vi "Bands_Main.vi"() -> ()   [LabVIEW 2024]
panel:
  out "Band sdev":dbl[][](graph)=[[0.3353772546826648, 0.4084966641388683, 0.5003856797342301, 0.6478785546391153], [0.24171080418296995, 0.35230228586245604, 0.3759732028560709, 0.5033028137104077], [0.22150470046762238, 0.3310214612014374, 0.36292977087510636, 0.4846104192263559], [0.19277937218238525, 0.3163483721041411, 0.36220368337093534, 0.46553114605932655], [0.19710471438384322, 0.32700679595860704, 0.3029446613190426, 0.4492463332131647], [0.16819270542381565, 0.31656348385339184, 0.35242193549705353, 0.427055332660449], [0.1730511001135913, 0.3123187705631996, 0.28252942293417965, 0.4121174290079004], [0.18605777226992246, 0.3065454715716774, 0.30903285463424796, 0.4641767502949591], [0.16818659712668763, 0.2724970239281444, 0.3555985592674683, 0.44590883736070325], [0.16166367655910485, 0.3076354897837717, 0.1949896816550948, 0.425321351327427], [0.14596500451769295, 0.2564716293467485, 0.3273362893696218, 0.44524121627082514], [0.1522592511319178, 0.29229701933526936, 0.22508584133149354, 0.44741414361442283], [0.14416764010644756, 0.28551749160160084, 0.27379096985814816, 0.4513185261438864], [0.17394046024499085, 0.27596830396614264, 0.3207441771446193, 0.451484391576808], [0.18167741119745937, 0.3045239509747764, 0.3000903307112586, 0.4481452184981623]]
  out "Band averages":dbl[][](graph)=[[8.680626893486426, 8.606188361284897, 12.33777384261614, 8.164276802226652], [8.632200271675586, 8.585758096325415, 12.307413887785566, 8.160446575120634], [8.624357532912756, 8.586135493161098, 12.319276005863179, 8.180110072455836], [8.616888139440022, 8.595026675175392, 12.33629120572369, 8.226922143493606], [8.616565415492165, 8.584035276166606, 12.32246082387115, 8.229027322702942], [8.62061301332379, 8.596221440305454, 12.351044023184894, 8.232899394943033], [8.617026039579283, 8.600839570954378, 12.356456884526148, 8.263498869003483], [8.624746125158572, 8.602677323174724, 12.37154176572413, 8.278567915663922], [8.612707346903331, 8.608183345601441, 12.400573947592072, 8.284231055046059], [8.610867167958734, 8.600263543620425, 12.357185805915336, 8.27523640312406], [8.60675426215495, 8.601551581496466, 12.40037793823958, 8.277235304213152], [8.613147504083752, 8.59805082398266, 12.383603489290671, 8.29105542356648], [8.621277473998088, 8.594195350754449, 12.433606127342339, 8.341301392017439], [8.617604109548608, 8.618650848461376, 12.428611676476121, 8.316097099348083], [8.635651626479794, 8.611122304003379, 12.453260394927339, 8.37908607476574]]
  in  "Bands 2":u16(ring)=2 items=["No Bands", "JC violin 200-7000 Flat (200-7000)", "JC violin (200-780-1740-2930-7000)", "JC violin (200-780-7000)", "MJ_Test (200-428-453-780-1740-2930-7000)"]
  in  "Files":path[](array[path])=[path "/Users/crogers/Dropbox (Rogers)/Violin Stuff/PC ViolnData/SoundCard2/SoundCard2 ModalShop7/Raw/SoundCard2 ModalShop7 H_001_001.wfm", path "/Users/crogers/Dropbox (Rogers)/Violin Stuff/PC ViolnData/SoundCard2/SoundCard2 ModalShop7/Raw/SoundCard2 ModalShop7 H_001_002.wfm", path "/Users/crogers/Dropbox (Rogers)/Violin Stuff/PC ViolnData/SoundCard2/SoundCard2 ModalShop7/Raw/SoundCard2 ModalShop7 H_001_003.wfm", path "/Users/crogers/Dropbox (Rogers)/Violin Stuff/PC ViolnData/SoundCard2/SoundCard2 ModalShop7/Raw/SoundCard2 ModalShop7 H_001_004.wfm", path "/Users/crogers/Dropbox (Rogers)/Violin Stuff/PC ViolnData/SoundCard2/SoundCard2 ModalShop7/Raw/SoundCard2 ModalShop7 H_001_005.wfm", path "/Users/crogers/Dropbox (Rogers)/Violin Stuff/PC ViolnData/SoundCard2/SoundCard2 ModalShop7/Raw/SoundCard2 ModalShop7 H_001_006.wfm", path "/Users/crogers/Dropbox (Rogers)/Violin Stuff/PC ViolnData/SoundCard2/SoundCard2 ModalShop7/Raw/SoundCard2 ModalShop7 H_001_007.wfm", path "/Users/crogers/Dropbox (Rogers)/Violin Stuff/PC ViolnData/SoundCard2/SoundCard2 ModalShop7/Raw/SoundCard2 ModalShop7 H_001_008.wfm", path "/Users/crogers/Dropbox (Rogers)/Violin Stuff/PC ViolnData/SoundCard2/SoundCard2 ModalShop7/Raw/SoundCard2 ModalShop7 H_001_009.wfm", path "/Users/crogers/Dropbox (Rogers)/Violin Stuff/PC ViolnData/SoundCard2/SoundCard2 ModalShop7/Raw/SoundCard2 ModalShop7 H_001_010.wfm", path "/Users/crogers/Dropbox (Rogers)/Violin Stuff/PC ViolnData/SoundCard2/SoundCard2 ModalShop7/Raw/SoundCard2 ModalShop7 H_002_001.wfm", path "/Users/crogers/Dropbox (Rogers)/Violin Stuff/PC ViolnData/SoundCard2/SoundCard2 ModalShop7/Raw/SoundCard2 ModalShop7 H_002_002.wfm", path "/Users/crogers/Dropbox (Rogers)/Violin Stuff/PC ViolnData/SoundCard2/SoundCard2 ModalShop7/Raw/SoundCard2 ModalShop7 H_002_003.wfm", path "/Users/crogers/Dropbox (Rogers)/Violin Stuff/PC ViolnData/SoundCard2/SoundCard2 ModalShop7/Raw/SoundCard2 ModalShop7 H_002_004.wfm", path "/Users/crogers/Dropbox (Rogers)/Violin Stuff/PC ViolnData/SoundCard2/SoundCard2 ModalShop7/Raw/SoundCard2 ModalShop7 H_002_005.wfm", path "/Users/crogers/Dropbox (Rogers)/Violin Stuff/PC ViolnData/SoundCard2/SoundCard2 ModalShop7/Raw/SoundCard2 ModalShop7 H_002_006.wfm", path "/Users/crogers/Dropbox (Rogers)/Violin Stuff/PC ViolnData/SoundCard2/SoundCard2 ModalShop7/Raw/SoundCard2 ModalShop7 H_002_007.wfm", path "/Users/crogers/Dropbox (Rogers)/Violin Stuff/PC ViolnData/SoundCard2/SoundCard2 ModalShop7/Raw/SoundCard2 ModalShop7 H_002_008.wfm", path "/Users/crogers/Dropbox (Rogers)/Violin Stuff/PC ViolnData/SoundCard2/SoundCard2 ModalShop7/Raw/SoundCard2 ModalShop7 H_002_009.wfm", path "/Users/crogers/Dropbox (Rogers)/Violin Stuff/PC ViolnData/SoundCard2/SoundCard2 ModalShop7/Raw/SoundCard2 ModalShop7 H_002_010.wfm", path "/Users/crogers/Dropbox (Rogers)/Violin Stuff/PC ViolnData/SoundCard2/SoundCard2 ModalShop7/Raw/SoundCard2 ModalShop7 H_003_001.wfm", path "/Users/crogers/Dropbox (Rogers)/Violin Stuff/PC ViolnData/SoundCard2/SoundCard2 ModalShop7/Raw/SoundCard2 ModalShop7 H_003_002.wfm", path "/Users/crogers/Dropbox (Rogers)/Violin Stuff/PC ViolnData/SoundCard2/SoundCard2 ModalShop7/Raw/SoundCard2 ModalShop7 H_003_003.wfm", path "/Users/crogers/Dropbox (Rogers)/Violin Stuff/PC ViolnData/SoundCard2/SoundCard2 ModalShop7/Raw/SoundCard2 ModalShop7 H_003_004.wfm", path "/Users/crogers/Dropbox (Rogers)/Violin Stuff/PC ViolnData/SoundCard2/SoundCard2 ModalShop7/Raw/SoundCard2 ModalShop7 H_003_005.wfm", path "/Users/crogers/Dropbox (Rogers)/Violin Stuff/PC ViolnData/SoundCard2/SoundCard2 ModalShop7/Raw/SoundCard2 ModalShop7 H_003_006.wfm", path "/Users/crogers/Dropbox (Rogers)/Violin Stuff/PC ViolnData/SoundCard2/SoundCard2 ModalShop7/Raw/SoundCard2 ModalShop7 H_003_007.wfm", path "/Users/crogers/Dropbox (Rogers)/Violin Stuff/PC ViolnData/SoundCard2/SoundCard2 ModalShop7/Raw/SoundCard2 ModalShop7 H_003_008.wfm", path "/Users/crogers/Dropbox (Rogers)/Violin Stuff/PC ViolnData/SoundCard2/SoundCard2 ModalShop7/Raw/SoundCard2 ModalShop7 H_003_009.wfm", path "/Users/crogers/Dropbox (Rogers)/Violin Stuff/PC ViolnData/SoundCard2/SoundCard2 ModalShop7/Raw/SoundCard2 ModalShop7 H_003_010.wfm", path "/Users/crogers/Dropbox (Rogers)/Violin Stuff/PC ViolnData/SoundCard2/SoundCard2 ModalShop7/Raw/SoundCard2 ModalShop7 H_004_001.wfm", path "/Users/crogers/Dropbox (Rogers)/Violin Stuff/PC ViolnData/SoundCard2/SoundCard2 ModalShop7/Raw/SoundCard2 ModalShop7 H_004_002.wfm", path "/Users/crogers/Dropbox (Rogers)/Violin Stuff/PC ViolnData/SoundCard2/SoundCard2 ModalShop7/Raw/SoundCard2 ModalShop7 H_004_003.wfm", path "/Users/crogers/Dropbox (Rogers)/Violin Stuff/PC ViolnData/SoundCard2/SoundCard2 ModalShop7/Raw/SoundCard2 ModalShop7 H_004_004.wfm", path "/Users/crogers/Dropbox (Rogers)/Violin Stuff/PC ViolnData/SoundCard2/SoundCard2 ModalShop7/Raw/SoundCard2 ModalShop7 H_004_005.wfm", path "/Users/crogers/Dropbox (Rogers)/Violin Stuff/PC ViolnData/SoundCard2/SoundCard2 ModalShop7/Raw/SoundCard2 ModalShop7 H_004_006.wfm", path "/Users/crogers/Dropbox (Rogers)/Violin Stuff/PC ViolnData/SoundCard2/SoundCard2 ModalShop7/Raw/SoundCard2 ModalShop7 H_004_007.wfm", path "/Users/crogers/Dropbox (Rogers)/Violin Stuff/PC ViolnData/SoundCard2/SoundCard2 ModalShop7/Raw/SoundCard2 ModalShop7 H_004_008.wfm", path "/Users/crogers/Dropbox (Rogers)/Violin Stuff/PC ViolnData/SoundCard2/SoundCard2 ModalShop7/Raw/SoundCard2 ModalShop7 H_004_009.wfm", path "/Users/crogers/Dropbox (Rogers)/Violin Stuff/PC ViolnData/SoundCard2/SoundCard2 ModalShop7/Raw/SoundCard2 ModalShop7 H_004_010.wfm", path "/Users/crogers/Dropbox (Rogers)/Violin Stuff/PC ViolnData/SoundCard2/SoundCard2 ModalShop7/Raw/SoundCard2 ModalShop7 H_005_001.wfm", path "/Users/crogers/Dropbox (Rogers)/Violin Stuff/PC ViolnData/SoundCard2/SoundCard2 ModalShop7/Raw/SoundCard2 ModalShop7 H_005_002.wfm", path "/Users/crogers/Dropbox (Rogers)/Violin Stuff/PC ViolnData/SoundCard2/SoundCard2 ModalShop7/Raw/SoundCard2 ModalShop7 H_005_003.wfm", path "/Users/crogers/Dropbox (Rogers)/Violin Stuff/PC ViolnData/SoundCard2/SoundCard2 ModalShop7/Raw/SoundCard2 ModalShop7 H_005_004.wfm", path "/Users/crogers/Dropbox (Rogers)/Violin Stuff/PC ViolnData/SoundCard2/SoundCard2 ModalShop7/Raw/SoundCard2 ModalShop7 H_005_005.wfm", path "/Users/crogers/Dropbox (Rogers)/Violin Stuff/PC ViolnData/SoundCard2/SoundCard2 ModalShop7/Raw/SoundCard2 ModalShop7 H_005_006.wfm", path "/Users/crogers/Dropbox (Rogers)/Violin Stuff/PC ViolnData/SoundCard2/SoundCard2 ModalShop7/Raw/SoundCard2 ModalShop7 H_005_007.wfm", path "/Users/crogers/Dropbox (Rogers)/Violin Stuff/PC ViolnData/SoundCard2/SoundCard2 ModalShop7/Raw/SoundCard2 ModalShop7 H_005_008.wfm", path "/Users/crogers/Dropbox (Rogers)/Violin Stuff/PC ViolnData/SoundCard2/SoundCard2 ModalShop7/Raw/SoundCard2 ModalShop7 H_005_009.wfm", path "/Users/crogers/Dropbox (Rogers)/Violin Stuff/PC ViolnData/SoundCard2/SoundCard2 ModalShop7/Raw/SoundCard2 ModalShop7 H_005_010.wfm", path "/Users/crogers/Dropbox (Rogers)/Violin Stuff/PC ViolnData/SoundCard2/SoundCard2 ModalShop8/Raw/SoundCard2 ModalShop8 H_001_001.wfm", path "/Users/crogers/Dropbox (Rogers)/Violin Stuff/PC ViolnData/SoundCard2/SoundCard2 ModalShop8/Raw/SoundCard2 ModalShop8 H_001_002.wfm", path "/Users/crogers/Dropbox (Rogers)/Violin Stuff/PC ViolnData/SoundCard2/SoundCard2 ModalShop8/Raw/SoundCard2 ModalShop8 H_001_003.wfm", path "/Users/crogers/Dropbox (Rogers)/Violin Stuff/PC ViolnData/SoundCard2/SoundCard2 ModalShop8/Raw/SoundCard2 ModalShop8 H_001_004.wfm", path "/Users/crogers/Dropbox (Rogers)/Violin Stuff/PC ViolnData/SoundCard2/SoundCard2 ModalShop8/Raw/SoundCard2 ModalShop8 H_001_005.wfm", path "/Users/crogers/Dropbox (Rogers)/Violin Stuff/PC ViolnData/SoundCard2/SoundCard2 ModalShop8/Raw/SoundCard2 ModalShop8 H_001_006.wfm", path "/Users/crogers/Dropbox (Rogers)/Violin Stuff/PC ViolnData/SoundCard2/SoundCard2 ModalShop8/Raw/SoundCard2 ModalShop8 H_001_007.wfm", path "/Users/crogers/Dropbox (Rogers)/Violin Stuff/PC ViolnData/SoundCard2/SoundCard2 ModalShop8/Raw/SoundCard2 ModalShop8 H_001_008.wfm", path "/Users/crogers/Dropbox (Rogers)/Violin Stuff/PC ViolnData/SoundCard2/SoundCard2 ModalShop8/Raw/SoundCard2 ModalShop8 H_001_009.wfm", path "/Users/crogers/Dropbox (Rogers)/Violin Stuff/PC ViolnData/SoundCard2/SoundCard2 ModalShop8/Raw/SoundCard2 ModalShop8 H_001_010.wfm", path "/Users/crogers/Dropbox (Rogers)/Violin Stuff/PC ViolnData/SoundCard2/SoundCard2 ModalShop8/Raw/SoundCard2 ModalShop8 H_002_001.wfm", path "/Users/crogers/Dropbox (Rogers)/Violin Stuff/PC ViolnData/SoundCard2/SoundCard2 ModalShop8/Raw/SoundCard2 ModalShop8 H_002_002.wfm", path "/Users/crogers/Dropbox (Rogers)/Violin Stuff/PC ViolnData/SoundCard2/SoundCard2 ModalShop8/Raw/SoundCard2 ModalShop8 H_002_003.wfm", path "/Users/crogers/Dropbox (Rogers)/Violin Stuff/PC ViolnData/SoundCard2/SoundCard2 ModalShop8/Raw/SoundCard2 ModalShop8 H_002_004.wfm", path "/Users/crogers/Dropbox (Rogers)/Violin Stuff/PC ViolnData/SoundCard2/SoundCard2 ModalShop8/Raw/SoundCard2 ModalShop8 H_002_005.wfm", path "/Users/crogers/Dropbox (Rogers)/Violin Stuff/PC ViolnData/SoundCard2/SoundCard2 ModalShop8/Raw/SoundCard2 ModalShop8 H_002_006.wfm", path "/Users/crogers/Dropbox (Rogers)/Violin Stuff/PC ViolnData/SoundCard2/SoundCard2 ModalShop8/Raw/SoundCard2 ModalShop8 H_002_007.wfm", path "/Users/crogers/Dropbox (Rogers)/Violin Stuff/PC ViolnData/SoundCard2/SoundCard2 ModalShop8/Raw/SoundCard2 ModalShop8 H_002_008.wfm", path "/Users/crogers/Dropbox (Rogers)/Violin Stuff/PC ViolnData/SoundCard2/SoundCard2 ModalShop8/Raw/SoundCard2 ModalShop8 H_002_009.wfm", path "/Users/crogers/Dropbox (Rogers)/Violin Stuff/PC ViolnData/SoundCard2/SoundCard2 ModalShop8/Raw/SoundCard2 ModalShop8 H_002_010.wfm", path "/Users/crogers/Dropbox (Rogers)/Violin Stuff/PC ViolnData/SoundCard2/SoundCard2 ModalShop8/Raw/SoundCard2 ModalShop8 H_003_001.wfm", path "/Users/crogers/Dropbox (Rogers)/Violin Stuff/PC ViolnData/SoundCard2/SoundCard2 ModalShop8/Raw/SoundCard2 ModalShop8 H_003_002.wfm", path "/Users/crogers/Dropbox (Rogers)/Violin Stuff/PC ViolnData/SoundCard2/SoundCard2 ModalShop8/Raw/SoundCard2 ModalShop8 H_003_003.wfm", path "/Users/crogers/Dropbox (Rogers)/Violin Stuff/PC ViolnData/SoundCard2/SoundCard2 ModalShop8/Raw/SoundCard2 ModalShop8 H_003_004.wfm", path "/Users/crogers/Dropbox (Rogers)/Violin Stuff/PC ViolnData/SoundCard2/SoundCard2 ModalShop8/Raw/SoundCard2 ModalShop8 H_003_005.wfm", path "/Users/crogers/Dropbox (Rogers)/Violin Stuff/PC ViolnData/SoundCard2/SoundCard2 ModalShop8/Raw/SoundCard2 ModalShop8 H_003_006.wfm", path "/Users/crogers/Dropbox (Rogers)/Violin Stuff/PC ViolnData/SoundCard2/SoundCard2 ModalShop8/Raw/SoundCard2 ModalShop8 H_003_007.wfm", path "/Users/crogers/Dropbox (Rogers)/Violin Stuff/PC ViolnData/SoundCard2/SoundCard2 ModalShop8/Raw/SoundCard2 ModalShop8 H_003_008.wfm", path "/Users/crogers/Dropbox (Rogers)/Violin Stuff/PC ViolnData/SoundCard2/SoundCard2 ModalShop8/Raw/SoundCard2 ModalShop8 H_003_009.wfm", path "/Users/crogers/Dropbox (Rogers)/Violin Stuff/PC ViolnData/SoundCard2/SoundCard2 ModalShop8/Raw/SoundCard2 ModalShop8 H_003_010.wfm", path "/Users/crogers/Dropbox (Rogers)/Violin Stuff/PC ViolnData/SoundCard2/SoundCard2 ModalShop8/Raw/SoundCard2 ModalShop8 H_004_001.wfm", path "/Users/crogers/Dropbox (Rogers)/Violin Stuff/PC ViolnData/SoundCard2/SoundCard2 ModalShop8/Raw/SoundCard2 ModalShop8 H_004_002.wfm", path "/Users/crogers/Dropbox (Rogers)/Violin Stuff/PC ViolnData/SoundCard2/SoundCard2 ModalShop8/Raw/SoundCard2 ModalShop8 H_004_003.wfm", path "/Users/crogers/Dropbox (Rogers)/Violin Stuff/PC ViolnData/SoundCard2/SoundCard2 ModalShop8/Raw/SoundCard2 ModalShop8 H_004_004.wfm", path "/Users/crogers/Dropbox (Rogers)/Violin Stuff/PC ViolnData/SoundCard2/SoundCard2 ModalShop8/Raw/SoundCard2 ModalShop8 H_004_005.wfm", path "/Users/crogers/Dropbox (Rogers)/Violin Stuff/PC ViolnData/SoundCard2/SoundCard2 ModalShop8/Raw/SoundCard2 ModalShop8 H_004_006.wfm", path "/Users/crogers/Dropbox (Rogers)/Violin Stuff/PC ViolnData/SoundCard2/SoundCard2 ModalShop8/Raw/SoundCard2 ModalShop8 H_004_007.wfm", path "/Users/crogers/Dropbox (Rogers)/Violin Stuff/PC ViolnData/SoundCard2/SoundCard2 ModalShop8/Raw/SoundCard2 ModalShop8 H_004_008.wfm", path "/Users/crogers/Dropbox (Rogers)/Violin Stuff/PC ViolnData/SoundCard2/SoundCard2 ModalShop8/Raw/SoundCard2 ModalShop8 H_004_009.wfm", path "/Users/crogers/Dropbox (Rogers)/Violin Stuff/PC ViolnData/SoundCard2/SoundCard2 ModalShop8/Raw/SoundCard2 ModalShop8 H_004_010.wfm", path "/Users/crogers/Dropbox (Rogers)/Violin Stuff/PC ViolnData/SoundCard2/SoundCard2 ModalShop8/Raw/SoundCard2 ModalShop8 H_005_001.wfm", path "/Users/crogers/Dropbox (Rogers)/Violin Stuff/PC ViolnData/SoundCard2/SoundCard2 ModalShop8/Raw/SoundCard2 ModalShop8 H_005_002.wfm", path "/Users/crogers/Dropbox (Rogers)/Violin Stuff/PC ViolnData/SoundCard2/SoundCard2 ModalShop8/Raw/SoundCard2 ModalShop8 H_005_003.wfm", path "/Users/crogers/Dropbox (Rogers)/Violin Stuff/PC ViolnData/SoundCard2/SoundCard2 ModalShop8/Raw/SoundCard2 ModalShop8 H_005_004.wfm", path "/Users/crogers/Dropbox (Rogers)/Violin Stuff/PC ViolnData/SoundCard2/SoundCard2 ModalShop8/Raw/SoundCard2 ModalShop8 H_005_005.wfm", path "/Users/crogers/Dropbox (Rogers)/Violin Stuff/PC ViolnData/SoundCard2/SoundCard2 ModalShop8/Raw/SoundCard2 ModalShop8 H_005_006.wfm", path "/Users/crogers/Dropbox (Rogers)/Violin Stuff/PC ViolnData/SoundCard2/SoundCard2 ModalShop8/Raw/SoundCard2 ModalShop8 H_005_007.wfm", path "/Users/crogers/Dropbox (Rogers)/Violin Stuff/PC ViolnData/SoundCard2/SoundCard2 ModalShop8/Raw/SoundCard2 ModalShop8 H_005_008.wfm", path "/Users/crogers/Dropbox (Rogers)/Violin Stuff/PC ViolnData/SoundCard2/SoundCard2 ModalShop8/Raw/SoundCard2 ModalShop8 H_005_009.wfm", path "/Users/crogers/Dropbox (Rogers)/Violin Stuff/PC ViolnData/SoundCard2/SoundCard2 ModalShop8/Raw/SoundCard2 ModalShop8 H_005_010.wfm"]
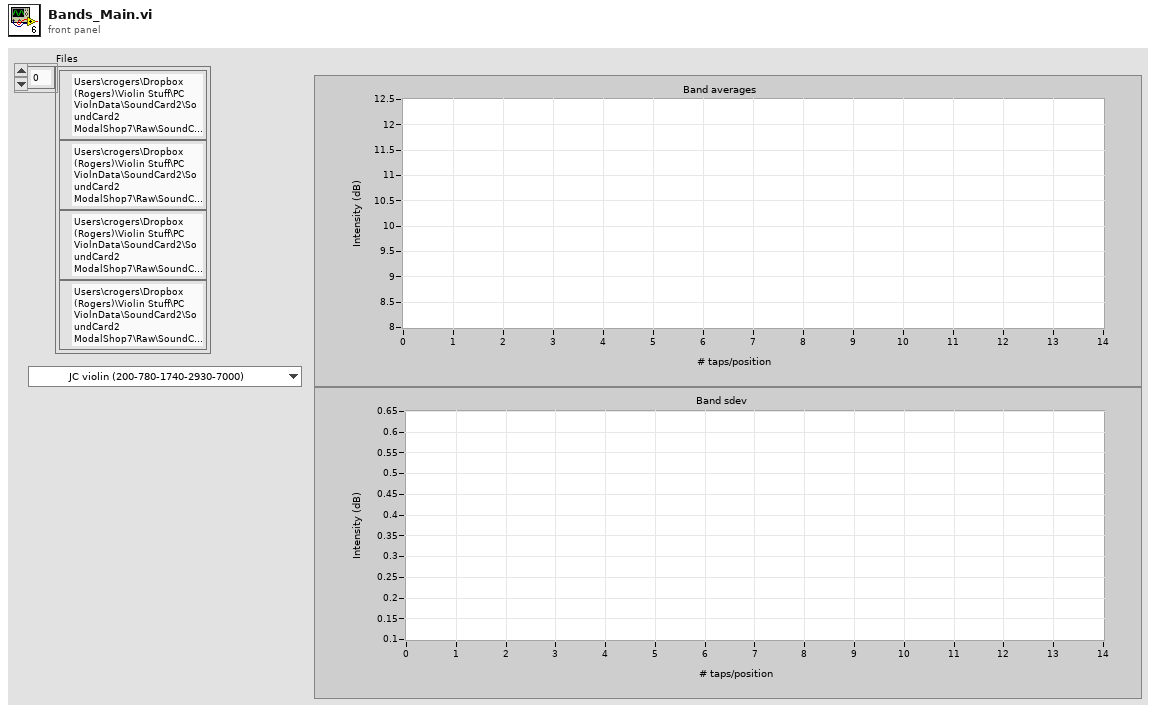
[diagram p1: front panel]
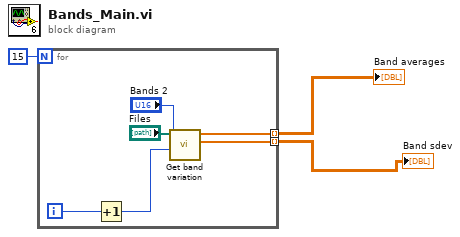
[diagram p0: block diagram]
diagram:
  n1 = for {
    N: 15 -> [_]
    tunnel: [w6] -> w2 mode=indexing
    tunnel: [w5] -> w1 mode=indexing
    i -> [w7]
    n2 = Increment(x=w7) -> (x+1=w4:i32)
    n3 = call "Get band variation.vi"("# taps / position"=w4, "Bands 2"="Bands 2", "Files"="Files") -> ("sdev"=w5:dbl[], "mean"=w6:dbl[])  [unwired: 7 in]
  }
  "Band averages" <- w2
  "Band sdev" <- w1
